vi "ControlOnConPane.vi"(8 "error in (no error)":errorcluster, 11 "Ctl Refnum":refnum<vi>) -> (0 "error out":errorcluster, 2 "Is connected to connector pane?":bool, 3 "Ctl Refnum out":refnum<vi>)   [LabVIEW 2020, in "NI_ReportGenerationCore.lvlib"]
uses:
  <vilib>/Utility/NIReport.llb/NI_ReportGenerationCore.lvlib
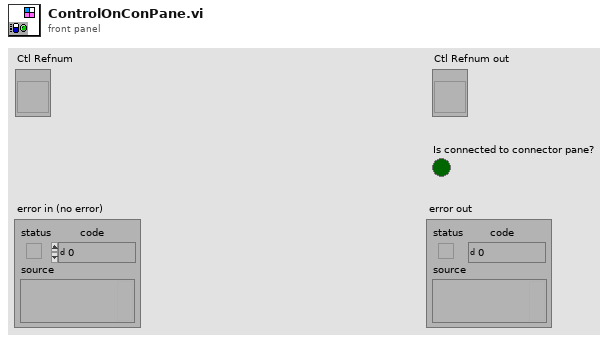
[diagram p1: front panel]
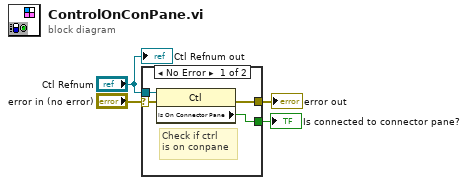
[diagram p0: block diagram]
diagram:
  n1 = case shown="No Error" "error in (no error)" {
    selector: "error in (no error)" -> [w8 w9]
    tunnel: [w7 w9] -> w3
    tunnel: "Ctl Refnum" -> [w6 _]
    tunnel: [w5 _] -> w2
    frame No Error {
      # "Check if ctrl\nis on conpane"
      n2 = property class="Ctl"(reference=w6, error in=w8) -> (error out=w7:errorcluster, "Is On Connector Pane"=w5:bool)  [unwired: 1 out]
    }
    frame Error {
    }
  }
  "error out" <- w3
  "Is connected to connector pane?" <- w2
  "Ctl Refnum out" <- "Ctl Refnum"
